vi "Wrap String in Quotes.vi"(1 "String in":string) -> (0 "String out":string)   [LabVIEW 2020, in "TALOS.lvlib" / "Run Utilities.lvlib"]
uses:
  Run Utilities.lvlib
  <vilib>/Utility/error.llb/Search and Replace Pattern.vi
  TALOS.lvlib
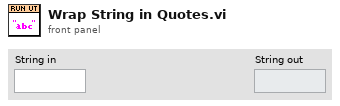
[diagram p1: front panel]
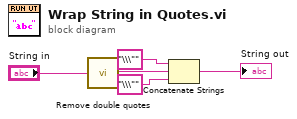
[diagram p0: block diagram]
diagram:
  n1 = call "Remove double quotes.vi"("Input string"="String in") -> ("Output string"=w5:string)  [unwired: 4 in]
  n2 = Concatenate Strings("\\\"" ("string"), w5, "\\\"" ("string")) -> (→"String out":string)
